vi "Pre-Build VI - Run Unit Tests.vi"(8 "error in (no error)":errorcluster) -> (0 "error out":errorcluster, 1 "VIs without test coverage":string[](array[string]), 2 "error type":enum16{"fatal", "non-fatal", "warning"}(ring))   [LabVIEW 2009]
uses:
  <userlib>/_OpenG.lib/array/array.llb/Conditional Auto-Indexing Tunnel (String)__ogtk.vi
  <userlib>/_OpenG.lib/array/array.llb/Empty 1D Array (String)__ogtk.vi
  <userlib>/_OpenG.lib/array/array.llb/Filter 1D Array (String)__ogtk.vi
panel:
  out "Failures":string[](array[string])
  in  "type specifier VI Refnum (for type only)":refnum<vi>
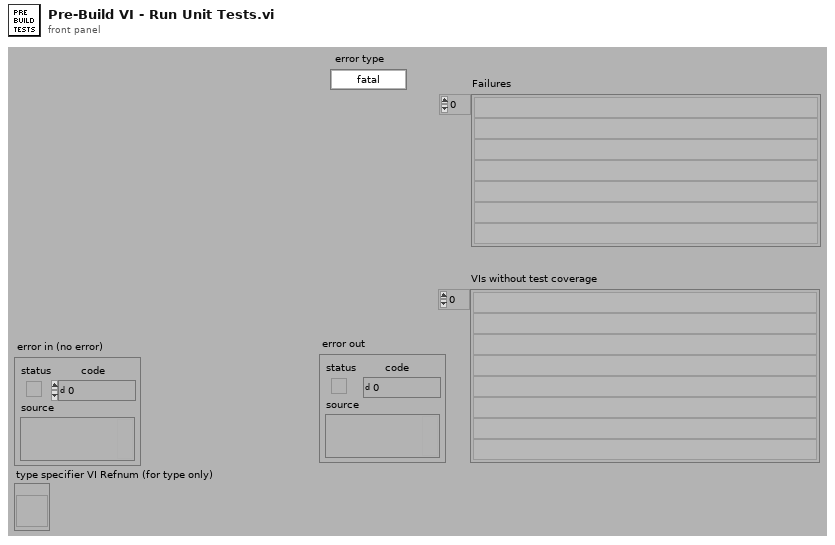
[diagram p1: front panel]
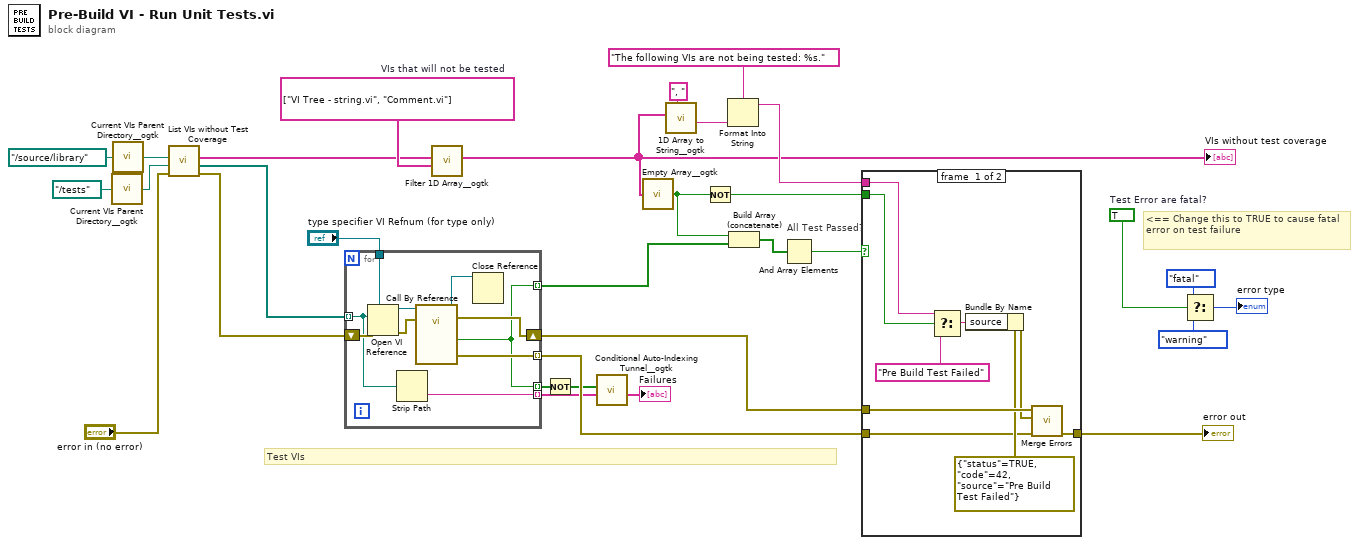
[diagram p0: block diagram]
diagram:
  w17 = TRUE  # Test Error are fatal?
  w29 = string[] ["VI Tree - string.vi", "Comment.vi"]  # VIs that will not be tested
  # "<== Change this to TRUE to cause fatal error on test failure"
  # "All Test Passed?"
  # "Test VIs"
  n1 = call <userlib>:"Current VIs Parent Directory__ogtk.vi"("Relative path (.)"=path "../tests") -> ("Parent Directory (+ Relative)"=w12:path)  [unwired: 4 in]
  n2 = call <userlib>:"Current VIs Parent Directory__ogtk.vi"("Relative path (.)"=path "../source/library") -> ("Parent Directory (+ Relative)"=w21:path)  [unwired: 4 in]
  n3 = call "List VIs without Test Coverage.vi"("error in (no error)"="error in (no error)", "Tests Root"=w12, "Source Root"=w21) -> ("error out"=w8:errorcluster, "Test VIs"=w11:path[], "VIs without test coverage"=w28:string[])  [unwired: 6 in]
  n4 = for {
    tunnel: w11 -> [w34] mode=indexing
    tunnel: "type specifier VI Refnum (for type only)" -> [w41]
    shift-right: [w38] -> w9
    shift-left: w8 -> [w37]
    tunnel: [w33] -> w7 mode=indexing
    tunnel: [w35] -> w6 mode=indexing
    tunnel: [w33] -> w4 mode=indexing
    tunnel: [w32] -> w2 mode=indexing
    n5 = Open VI Reference(type specifier VI Refnum (for type only)=w41, vi path=w34, error in (no error)=w37) -> (vi reference=w40:refnum<vi>, error out=w39:errorcluster)  [unwired: 3 in]
    n6 = Strip Path(path=w34) -> (name=w32:string)  [unwired: 1 out]
    n7 = call-by-ref "?"(reference=w40, error in=w39) -> (reference out=w36:refnum<vi>, error out=w38:errorcluster, 0:"error out"=w35:errorcluster, "pass"=w33:bool)  [unwired: 10 in]
    n8 = Close Reference(reference=w36) -> ()  [unwired: 1 in, 1 out]
  }
  n9 = call-poly <userlib>:"Filter 1D Array__ogtk.vi"("items to filter"=w29, "array"=w28) -> ("filtered array"=w5:string[])  [unwired: 4 in, 1 out]
  "VIs without test coverage" <- w5
  n10 = Not(x=w4) -> (.not. x?=w3:bool[])
  n11 = call-poly <userlib>:"Conditional Auto-Indexing Tunnel__ogtk.vi"("Array in"=w2, "Elements to keep"=w3) -> ("Filtered Array out"=→"Failures":string[])  [unwired: 5 in]
  n12 = call-poly <userlib>:"Empty Array__ogtk.vi"("Array"=w5) -> ("Empty Array?"=w23:bool)  [unwired: 8 in]
  n13 = call <userlib>:"1D Array to String__ogtk.vi"("delimiter (Tab)"=", ", "Array of Strings"=w5) -> ("delimited string"=w26:string)  [unwired: 9 in]
  n14 = Not(x=w23) -> (.not. x?=w22:bool)
  n15 = Format Into String(format string="The following VIs are not being tested: %s.", w26) -> (resulting string=w24:string)  [unwired: 2 in, 1 out]
  n16 = Build Array (concatenate)(w23, w7) -> (w31:bool[])
  n17 = And Array Elements(Boolean array=w31) -> (logical AND=w30:bool)
  n18 = case shown="False" w30 {
    tunnel: w9 -> [w50 w51]
    tunnel: [w49 w51] -> w19
    tunnel: w22 -> [w48 _]
    tunnel: w24 -> [w47 _]
    tunnel: w6 -> [w42 _]
    frame #0 {
      n19 = Select(t=w47, s=w48, f="Pre Build Test Failed" ("source")) -> (s? t:f=w45:string)
      n20 = Bundle By Name(cluster=errorcluster {"status"=TRUE, "code"=42, "source"="Pre Build Test Failed"} ("error out"), "source"=w45) -> (w44:errorcluster)
      n21 = call <vilib>:"Merge Errors.vi"("error array in"=w42, "error in 2 (no error)"=w44, "error in 1 (no error)"=w50) -> ("error out"=w49:errorcluster)  [unwired: 4 in]
    }
    frame #1 {
    }
  }
  "error out" <- w19
  n22 = Select(t=enum16{"fatal", "non-fatal", "warning"}."fatal" ("error type"), s=w17, f=enum16{"fatal", "non-fatal", "warning"}."warning" ("error type")) -> (s? t:f=→"error type":enum16{"fatal", "non-fatal", "warning"})
